vi "Follow Trajectory.vi"(1 "Time After Done[sec]":dbl, 2 "Drive Name":string="Drive", 3 "Motion Profile":T1(array[cluster])) -> ()   [LabVIEW 2016]
uses:
  Sensors/Navx/navX Library v2/navX Library v2.lvlib
  <vilib>/addons/control/pid/NI_PID_pid.lvlib
  Robot Global Data.vi
  <vilib>/addons/control/pid/pid.llb/PID Control Input Filter (DBL).vi
panel:
  out "x+y":dbl
  out "coerced(x)":dbl
  in  "FF Deadzone Comp":dbl
  out "Distance L":dbl
  out "Distance R":dbl
  out "Robot Position":cluster{dbl[], dbl[]}[](graph)
  out "Angle Error":dbl(graph)
  out "New Angle Out":dbl
  in  "Kv":dbl=-0.008
  in  "Ka":dbl
  out "element":T2
  in  "Drive PID Gains":cluster{"Kp":dbl, "Ki":dbl, "Kd":dbl}={"Kp"=-0.3, "Ki"=0.0, "Kd"=0.0}
  in  "Angle PID Gains":cluster{"Kp":dbl, "Ki":dbl, "Kd":dbl}={"Kp"=0.1, "Ki"=0.0, "Kd"=0.0}
  out "Distance* Error":dbl(graph)
  out "Total Time":dbl
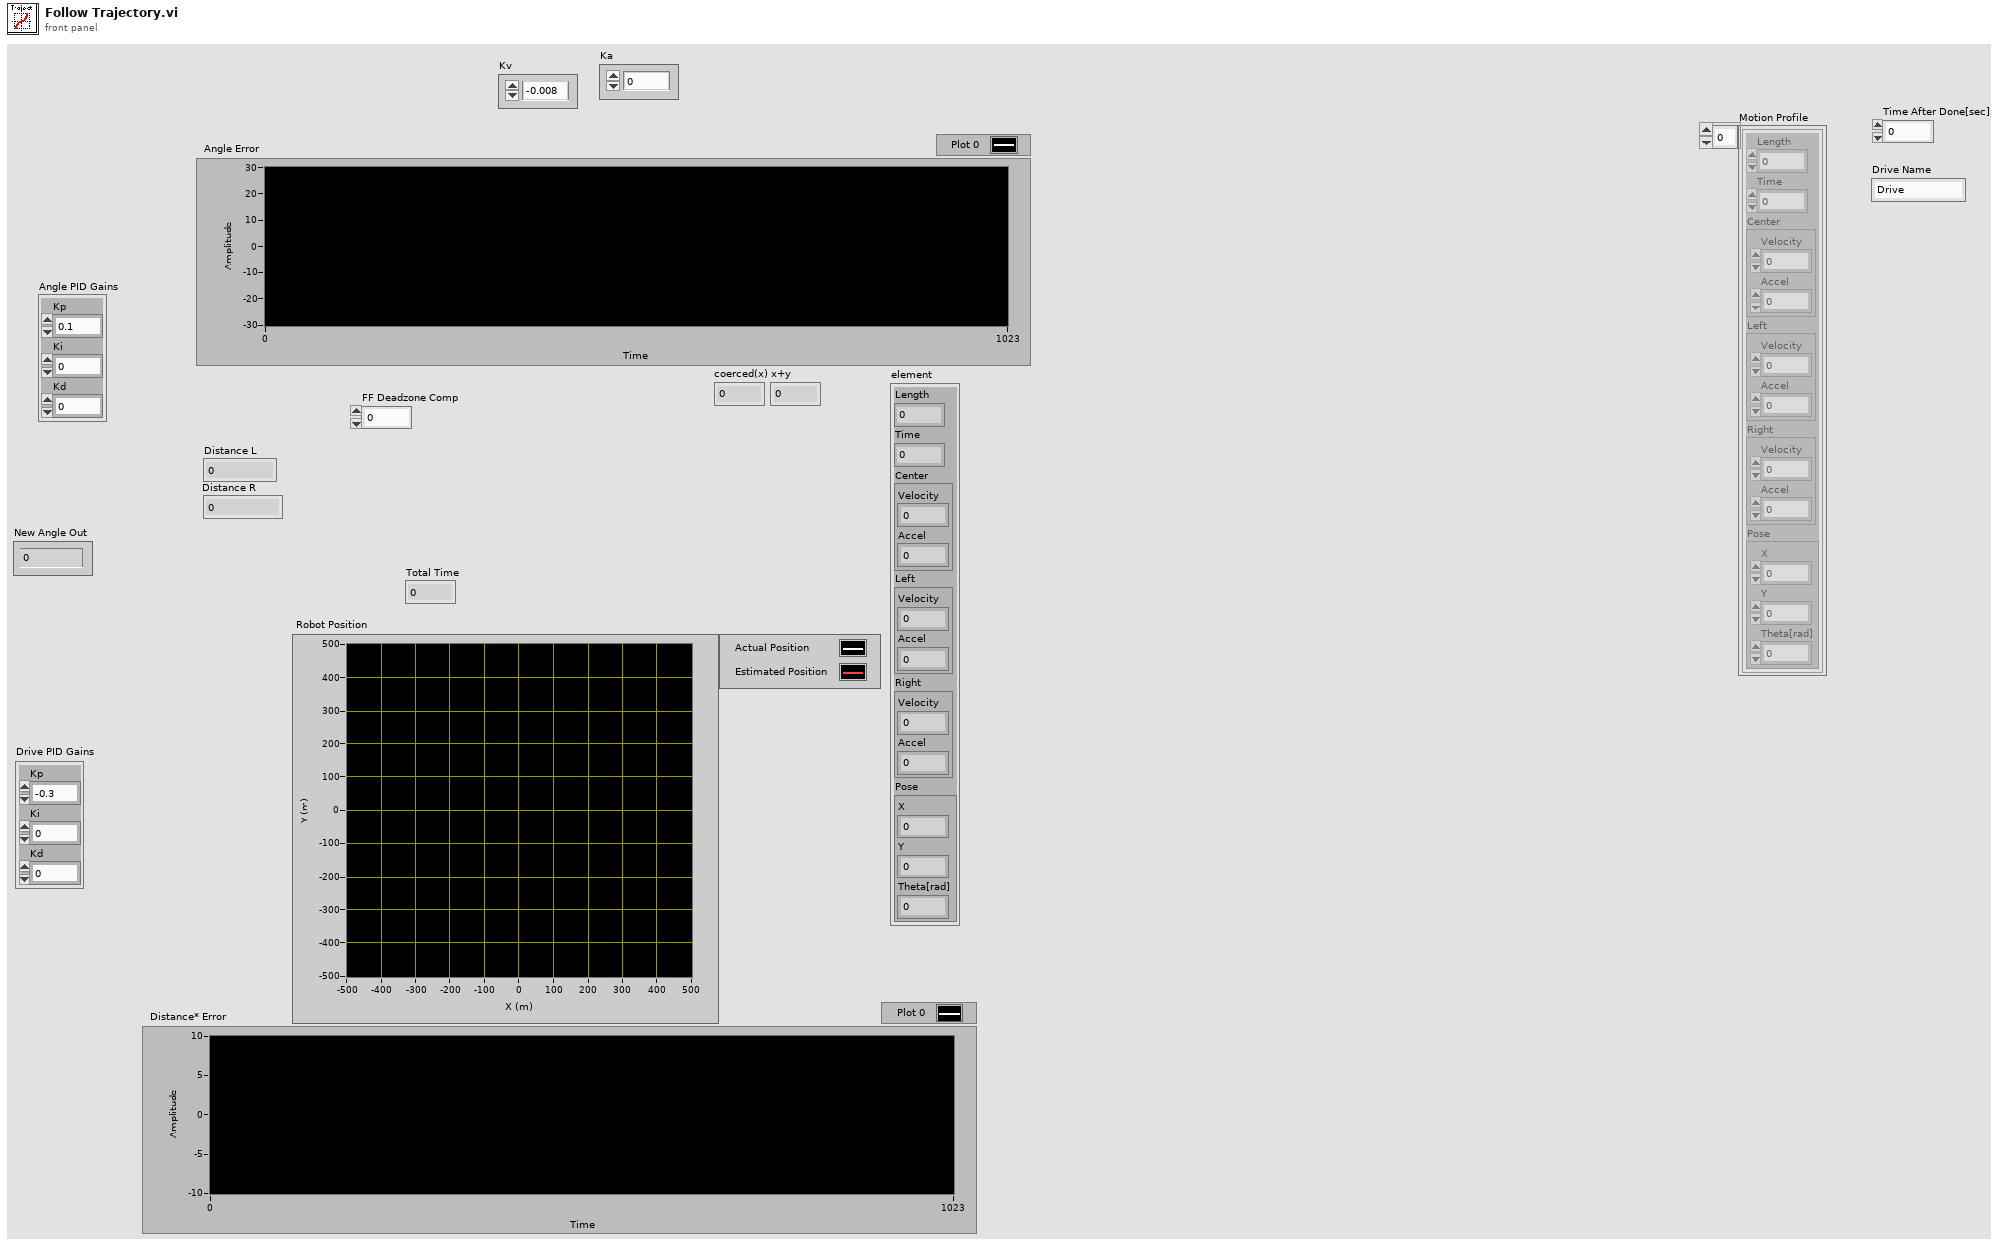
[diagram p1: front panel]
types:
  T1 = cluster{"Length":dbl, "Time":dbl, "Center":cluster{"Velocity":dbl, "Accel":dbl}, "Left":cluster{"Velocity":dbl, "Accel":dbl}, "Right":cluster{"Velocity":dbl, "Accel":dbl}, "Pose":cluster{"X":dbl, "Y":dbl, "Theta[rad]":dbl}}[]
  T2 = cluster{"Length":dbl, "Time":dbl, "Center":cluster{"Velocity":dbl, "Accel":dbl}, "Left":cluster{"Velocity":dbl, "Accel":dbl}, "Right":cluster{"Velocity":dbl, "Accel":dbl}, "Pose":cluster{"X":dbl, "Y":dbl, "Theta[rad]":dbl}}
  T3 = cluster{"Yaw":dbl, "Roll":dbl, "Pitch":dbl, "Heading":dbl, "Fused Heading":dbl}
  T4 = typedef "WPI_EncoderDevRef.ctl" = cluster{"DevStatus":errorcluster, "EncoderIndex":T5, "CounterIndex":T6, "DistancePerCount":dbl, "Decoding Type":T7}
  T5 = typedef "FPGA_EncoderIdx.ctl" = enum8{"Enc 0", "Enc 1", "Enc 2", "Enc 3", "Enc 4", "Enc 5", "Enc 6", "Enc 7", "Invalid"}
  T6 = typedef "FPGA_CounterCtrSystemIndex.ctl" = enum8{"Ctr 0", "Ctr 1", "Ctr 2", "Ctr 3", "Ctr 4", "Ctr 5", "Ctr 6", "Ctr 7", "Invalid"}
  T7 = typedef "WPI_EncoderType.ctl" = enum16{"1x", "2x", "4x"}
  T8 = typedef "WPI_RobotDriveDevRef.ctl" = cluster{"DevStatus":errorcluster, "Motors[]":T9[], "Square Inputs":bool, "Max Output":dbl}
  T9 = typedef "WPI_MotorControlDeviceRef.ctl" = cluster{"DeviceStatus":errorcluster, "Type":T10, "PWM":cluster{"PWM Channel":T11, "DeadBand":T12}, "CAN":cluster{"Device Number":u8, "SetOutput VI Ref":variant, "GetOutput VI Ref":variant, "Enable VI Ref":variant, "Disable VI Ref":variant, "Data":variant}, "Invert":bool}
  T10 = typedef "WPI_MotorControlType.ctl" = enum16{"PWM", "CAN"}
  T11 = typedef "FPGA_DIOPWMChannel.ctl" = enum8{"PWM 0", "PWM 1", "PWM 2", "PWM 3", "PWM 4", "PWM 5", "PWM 6", "PWM 7", "PWM 8", "PWM 9", "PWM MXP 0", "PWM MXP 1", "PWM MXP 2", "PWM MXP 3", "PWM MXP 4", "PWM MXP 5", "PWM MXP 6", "PWM MXP 7", "PWM MXP 8", "PWM MXP 9", "Invalid"}
  T12 = typedef "WPI_PWMDeadband.ctl" = cluster{"Name":string, "maxPositivePwm":i32, "minPositivePwm":i32, "centerPwm":i32, "maxNegativePwm":i32, "minNegativePwm":i32, "angularRange":u16}
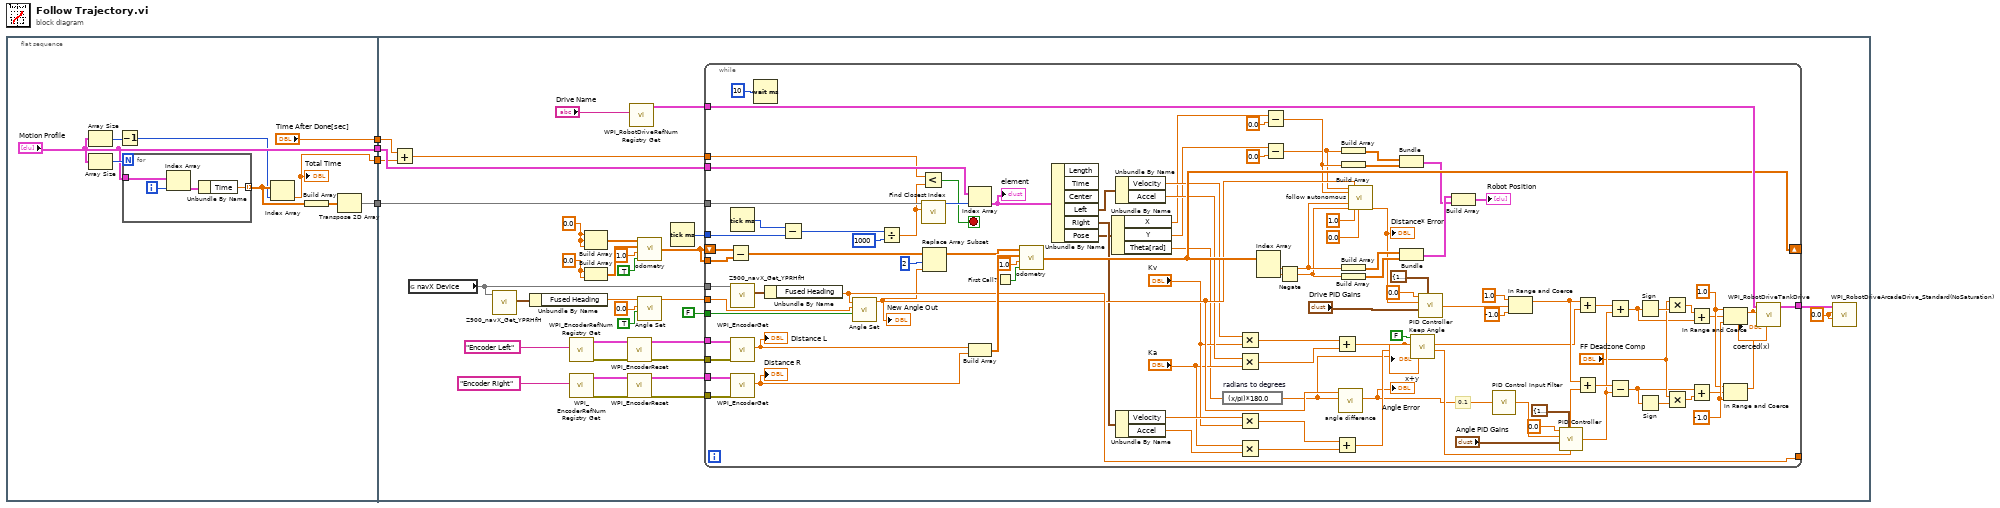
[diagram p0: block diagram]
diagram:
  n1 = flat-sequence {
    tunnel: [w11] -> w4
    tunnel: ["Motion Profile"] -> w3
    tunnel: [w6] -> w2
    tunnel: ["Time After Done[sec]"] -> w1
    tunnel: w4 -> [w23]
    tunnel: w3 -> [w22]
    tunnel: w2 -> [w19]
    tunnel: w1 -> [w20]
    frame #0 {
      n2 = Array Size(array="Motion Profile") -> (size(s)=w7:i32)
      n3 = Array Size(array="Motion Profile") -> (size(s)=w13:i32)
      n4 = Decrement(x=w7) -> (x-1=w8:i32)
      n5 = for {
        N: w13 -> [_]
        tunnel: "Motion Profile" -> [w17]
        tunnel: [w14] -> w10 mode=indexing
        i -> [w16]
        n6 = Index Array(array=w17, index=w16) -> (element=w15:T2)
        n7 = Unbundle By Name(w15) -> ("Time"=w14:dbl)
      }
      n8 = Index Array(array=w10, index=w8) -> (element=w6:dbl)
      "Total Time" <- w6
      n9 = Build Array(w10) -> (w12:dbl[][])
      n10 = Transpose 2D Array(2D array=w12) -> (transposed array=w11:dbl[][])
    }
    frame #1 {
      w45 = 0.0 ("element")
      w46 = 0.0 ("element")
      w47 = 0.0 ("Y axis value")
      n11 = Add(x=w20, y=w19) -> (x+y=w18:dbl)
      n12 = global read "Robot Global Data.vi" "navX Device"() -> (w24)
      n13 = call "Z900_navX_Get_YPRHfH.vi"("navX Device"=w24) -> ("YRPHfH"=w29:T3)  [unwired: 7 in, 3 out]
      n14 = Unbundle By Name(w29) -> ("Fused Heading"=w27:dbl)
      n15 = call <vilib>:"WPI_EncoderRefNum Registry Get.vi"("refnum name"="Encoder Left") -> ("error out"=w39:errorcluster, "EncoderDevRef"=w38:T4)  [unwired: 9 in]
      n16 = call <vilib>:"WPI_EncoderRefNum Registry Get.vi"("refnum name"="Encoder Right") -> ("error out"=w37:errorcluster, "EncoderDevRef"=w36:T4)  [unwired: 9 in]
      n17 = Build Array(w46, w46, w46) -> (w31:dbl[])
      n18 = Build Array(w45, w45) -> (w44:dbl[])
      n19 = call <vilib>:"WPI_EncoderReset.vi"("error in (no error)"=w39, "EncoderDevRef"=w38) -> ("error out"=w34:errorcluster, "EncoderDevRef"=w35:T4)  [unwired: 8 in]
      n20 = call <vilib>:"WPI_EncoderReset.vi"("error in (no error)"=w37, "EncoderDevRef"=w36) -> ("error out"=w32:errorcluster, "EncoderDevRef"=w33:T4)  [unwired: 8 in]
      n21 = call <vilib>:"WPI_RobotDriveRefNum Registry Get.vi"("refnum name"="Drive Name") -> ("RobotDriveDevRef"=w49:T8)  [unwired: 1 in, 9 out]
      n22 = call "odometry.vi"("reset"=TRUE, "distance between sides of wheels"=1.0, "encoders in"=w44, "state in"=w31) -> ("state out"=w21:dbl[])
      n23 = call "Angle Set.vi"("Set Angle?"=TRUE, "Angle Set"=0.0, "Angle In"=w27) -> ("New Angle Out"=w26:dbl)  [unwired: 8 in]
      n24 = Tick Count (ms)() -> (millisecond timer value=w51:u32)
      n25 = while {
        tunnel: w51 -> [w152]
        tunnel: w49 -> [w135]
        tunnel: [w134] -> w48
        shift-right: [w128] -> _
        shift-left: w21 -> [w67]
        tunnel: w35 -> [w139]
        tunnel: w34 -> [w138]
        tunnel: w33 -> [w137]
        tunnel: w32 -> [w136]
        tunnel: [w118] -> _
        tunnel: w26 -> [w126]
        tunnel: FALSE ("Set Angle?") -> [w125]
        tunnel: w24 -> [w119]
        tunnel: w23 -> [w109]
        tunnel: w22 -> [w107]
        tunnel: w21 -> [w66]
        tunnel: w18 -> [w64]
        stop <- w62 stop-if-true
        w127 = -1.0 ("lower limit")
        w124 = 1.0 ("upper limit")
        # "0.1"
        n26 = Subtract(x=w67, y=w66) -> (x-y=w65:dbl[])
        n27 = Tick Count (ms)() -> (millisecond timer value=w151:u32)
        n28 = call "Z900_navX_Get_YPRHfH.vi"("navX Device"=w119) -> ("YRPHfH"=w120:T3)  [unwired: 7 in, 3 out]
        n29 = call <vilib>:"WPI_EncoderGet.vi"("error in (no error)"=w138, "EncoderDevRef"=w139) -> ("Distance"=w116:dbl)  [unwired: 4 in, 5 out]
        "Distance L" <- w116
        n30 = call <vilib>:"WPI_EncoderGet.vi"("error in (no error)"=w136, "EncoderDevRef"=w137) -> ("Distance"=w115:dbl)  [unwired: 4 in, 5 out]
        "Distance R" <- w115
        n31 = Wait (ms)(milliseconds to wait=u32 10) -> ()  [unwired: 1 out]
        n32 = Unbundle By Name(w120) -> ("Fused Heading"=w118:dbl)
        n33 = Subtract(x=w151, y=w152) -> (x-y=w85:u32)
        n34 = call "Angle Set.vi"("Set Angle?"=w125, "Angle Set"=w126, "Angle In"=w118) -> ("New Angle Out"=w117:dbl)  [unwired: 8 in]
        "New Angle Out" <- w117
        n35 = Divide(x=w85, y=u32 1000) -> (x/y=w63:dbl)
        n36 = Less?(x=w64, y=w63) -> (x < y?=w62:bool)
        n37 = call "Find Closest Index.vi"("Time"=w63, "Array"=w109) -> ("Index"=w108:i32)  [unwired: 9 in]
        n38 = Replace Array Subset(array=w65, new element=w117, index=2) -> (w143:dbl[])
        n39 = Index Array(array=w107, index=w108) -> (element=w106:T2)
        "element" <- w106
        n40 = Build Array(w116, w115) -> (w149:dbl[])
        n41 = First Call?() -> (First Call?: T/F=w140:bool)
        n42 = call "odometry.vi"("reset"=w140, "distance between sides of wheels"=1.0, "encoders in"=w149, "state in"=w143) -> ("state out"=w128:dbl[])
        n43 = Unbundle By Name(w106) -> ("Left"=w105:cluster{"Velocity":dbl, "Accel":dbl}, "Right"=w104:cluster{"Velocity":dbl, "Accel":dbl}, "Pose"=w90:cluster{"X":dbl, "Y":dbl, "Theta[rad]":dbl})  [unwired: 3 out]
        n44 = Unbundle By Name(w90) -> ("X"=w81:dbl, "Y"=w80:dbl, "Theta[rad]"=w89:dbl)
        n45 = Unbundle By Name(w105) -> ("Velocity"=w103:dbl, "Accel"=w102:dbl)
        n46 = Unbundle By Name(w104) -> ("Velocity"=w97:dbl, "Accel"=w94:dbl)
        n47 = expression code="(x/pi)*180.0" "radians to degrees"(w89) -> (w88:dbl)
        n48 = Multiply(x=w103, y="Kv") -> (x*y=w100:dbl)
        n49 = Multiply(x=w102, y="Ka") -> (x*y=w101:dbl)
        n50 = Multiply(x=w97, y="Kv") -> (x*y=w99:dbl)
        n51 = Multiply(x="Ka", y=w94) -> (x*y=w98:dbl)
        n52 = Index Array(array=w128) -> (element #1=w83:dbl, element #2=w145:dbl)  [unwired: 2 in]
        n53 = Subtract(x=w81, y=0.0) -> (x-y=w112:dbl)
        n54 = Subtract(x=w80, y=0.0) -> (x-y=w82:dbl)
        n55 = Negate(x=w145) -> (-x=w52:dbl)
        n56 = Add(x=w100, y=w101) -> (x+y=w93:dbl)
        "x+y" <- w93
        n57 = Add(x=w99, y=w98) -> (x+y=w91:dbl)
        n58 = call "angle difference.vi"("angle2"=w88, "angle1"=w117) -> ("angle diff"=w70:dbl)  [unwired: 9 in]
        "Angle Error" <- w70
        n59 = Build Array(w82) -> (w123:dbl[])
        n60 = Build Array(w112) -> (w122:dbl[])
        n61 = Build Array(w83) -> (w147:dbl[])
        n62 = Build Array(w52) -> (w148:dbl[])
        n63 = call "follow autonomous.vi"("x"=w82, "y"=w112, "robot x"=w83, "robot y"=w52, "robot angle"=w117, "speed kp"=1.0, "v"=0.0) -> ("newV"=w68:dbl)  [unwired: 12 in]
        "Distance* Error" <- w68
        n64 = Bundle(w123, w122) -> (w121:cluster{dbl[], dbl[]})  [unwired: 1 in]
        n65 = Bundle(w147, w148) -> (w146:cluster{dbl[], dbl[]})  [unwired: 1 in]
        n66 = call "Keep Angle.vi"("Angle"=w88, "Right Speed"=w91, "Left Speed"=w93, "Keep Angle"=FALSE) -> ("Right"=w113:dbl, "Left"=w114:dbl)  [unwired: 6 in]
        n67 = call "PID Controller.vi"("setpoint"=0.0, "process variable"=w68, "PID Gains"="Drive PID Gains", "Constrain"=cluster{"Max Control":dbl, "Min Control":dbl} {"Max Control"=1.0, "Min Control"=-1.0}) -> ("Control Signal"=w71:dbl)  [unwired: 1 in]
        n68 = Build Array(w146, w121) -> (→"Robot Position":cluster{dbl[], dbl[]}[])
        n69 = call-poly <vilib>:"PID Control Input Filter.vi"("input"=w70) -> ("output"=w69:dbl)  [unwired: 4 in]
        n70 = In Range and Coerce(upper limit=1.0, x=w71, lower limit=-1.0) -> (coerced(x)=w131:dbl)  [unwired: 1 out]
        n71 = call "PID Controller.vi"("setpoint"=0.0, "process variable"=w69, "PID Gains"="Angle PID Gains", "Constrain"=cluster{"Max Control":dbl, "Min Control":dbl} {"Max Control"=1.0, "Min Control"=-1.0}) -> ("Control Signal"=w73:dbl)  [unwired: 1 in]
        n72 = Add(x=w131, y=w114) -> (x+y=w133:dbl)
        n73 = Add(x=w131, y=w113) -> (x+y=w132:dbl)
        n74 = Add(x=w133, y=w73) -> (x+y=w54:dbl)
        n75 = Subtract(x=w132, y=w73) -> (x-y=w57:dbl)
        n76 = Sign(1:w54) -> (0:w61:dbl)
        n77 = Sign(1:w57) -> (0:w60:dbl)
        n78 = Multiply(x="FF Deadzone Comp", y=w61) -> (x*y=w55:dbl)
        n79 = Multiply(x="FF Deadzone Comp", y=w60) -> (x*y=w58:dbl)
        n80 = Add(x=w55, y=w54) -> (x+y=w53:dbl)
        n81 = Add(x=w57, y=w58) -> (x+y=w56:dbl)
        n82 = In Range and Coerce(upper limit=w124, x=w53, lower limit=w127) -> (coerced(x)=w111:dbl)  [unwired: 1 out]
        "coerced(x)" <- w111
        n83 = In Range and Coerce(upper limit=w124, x=w56, lower limit=w127) -> (coerced(x)=w110:dbl)  [unwired: 1 out]
        n84 = call <vilib>:"WPI_RobotDriveTankDrive.vi"("Right axis value"=w110, "Left axis value"=w111, "RobotDriveDevRef"=w135) -> ("RobotDriveDevRef"=w134:T8)  [unwired: 6 in, 2 out]
      }
      n85 = call <vilib>:"WPI_RobotDriveArcadeDrive_Standard(NoSaturation).vi"("Y axis value"=w47, "X axis value"=w47, "RobotDriveDevRef"=w48) -> ()  [unwired: 1 in, 8 out]
    }
  }
